vi "Rotate xy.vi"(0 "In y":dbl, 3 "In x":dbl, 4 "Rotate degrees":dbl) -> (5 "Out y":dbl, 6 "Out x":dbl)   [LabVIEW 2023]
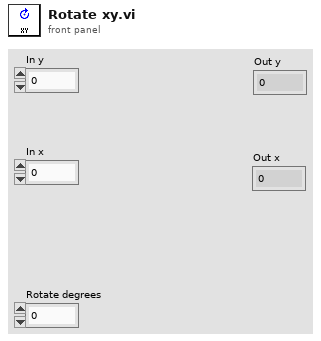
[diagram p1: front panel]
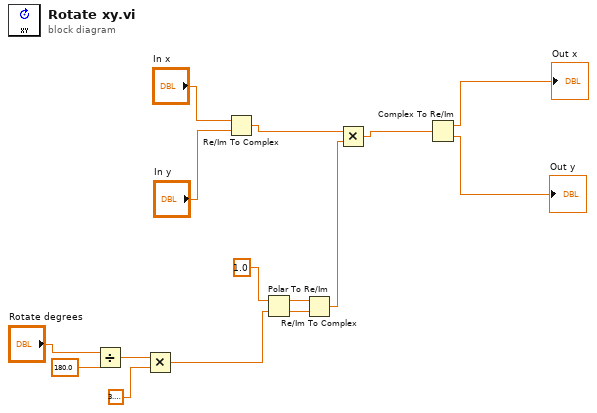
[diagram p0: block diagram]
diagram:
  n1 = Divide(x="Rotate degrees", y=180.0) -> (x/y=w9:dbl)
  n2 = Multiply(x=w9, y=3.141592653589793) -> (x*y=w8:dbl)
  n3 = Re/Im To Complex(1:"In y", 2:"In x") -> (0:w5:cdb)
  n4 = Polar To Re/Im(2:w8, 3:1.0 ("r")) -> (0:w6:dbl, 1:w7:dbl)
  n5 = Re/Im To Complex(1:w6, 2:w7) -> (0:w4:cdb)
  n6 = Multiply(x=w5, y=w4) -> (x*y=w3:cdb)
  n7 = Complex To Re/Im(x + iy=w3) -> (x=→"Out x":dbl, y=→"Out y":dbl)
